vi "svfa_Check Data Valid [Nx1 Dual FFT].vi"(0 "stimulus signal X [EUx]":waveform(dbl), 1 "response signals Y [EUy]":waveform(dbl)[](array[waveform]), 2 "window":T3=1 items=["None"=0, "Hanning"=1, "Hamming"=2, "Blackman-Harris"=3, "Exact Blackman"=4, "Blackman"=5, "Flat Top"=6, "4 Term B-Harris "=7, "7 Term B-Harris"=8, "Low Sidelobe"=9, "Force - Exponential"=10, "Blackman Nuttall"=11, "Triangle"=30, "Bartlett-Hanning"=31, "Bohman"=32, "Parzen"=33, "Welch"=34, "Kaiser"=60, "Dolph-Chebyshev"=61, "Gaussian"=62], 3 "force/exp settings":T2={"force window [%]"=50.0, "exp window [%]"=10.0} {"exp window [%]" min=0.0 max=100.0 format="%.2f"; "force window [%]" min=0.0 max=100.0 format="%.2f"}, 4 "averaging parameters":T5={"averaging mode"=enum."No averaging", "weighting mode"=enum."Linear", "number of averages"=10, "linear mode"=enum."Auto restart"}, 5 "error in (no error)":errorcluster, 7 "processing control in":T4(ring), 8 "restart averaging (F)":bool, 9 "FRF mode":enum16{"H1", "H2", "H3"}(ring), 10 "measurement":T1(ring)=enum."Frequency response") -> (11 "dup FRF mode":enum16{"H1", "H2", "H3"}(ring), 13 "processing control out":T4(ring), 14 "dup stimulus signal X [EUx]":waveform(dbl), 15 "dup response signals Y [EUy]":waveform(dbl)[](array[waveform]), 16 "window":T3=1 items=["None"=0, "Hanning"=1, "Hamming"=2, "Blackman-Harris"=3, "Exact Blackman"=4, "Blackman"=5, "Flat Top"=6, "4 Term B-Harris "=7, "7 Term B-Harris"=8, "Low Sidelobe"=9, "Force - Exponential"=10, "Blackman Nuttall"=11, "Triangle"=30, "Bartlett-Hanning"=31, "Bohman"=32, "Parzen"=33, "Welch"=34, "Kaiser"=60, "Dolph-Chebyshev"=61, "Gaussian"=62], 17 "dup force/exp settings":T2={"force window [%]"=50.0, "exp window [%]"=10.0} {"exp window [%]" min=0.0 max=100.0 format="%.2f"; "force window [%]" min=0.0 max=100.0 format="%.2f"}, 18 "dup averaging parameters":T5={"averaging mode"=enum."No averaging", "weighting mode"=enum."Linear", "number of averages"=10, "linear mode"=enum."Auto restart"}, 19 "error out":errorcluster)   [LabVIEW 2017]
uses:
  <vilib>/addons/_NISVFA/_Shared subVIs/Controls/svc_Window [Dual FFT].ctl
  <vilib>/addons/_NISVFA/_Shared subVIs/Common/svc_Check for Waveform Parameter Continuity (N Ch).vi
  <vilib>/addons/_NISVFA/_Shared subVIs/Common/svc_Check for Waveform Parameter Continuity (1 Ch).vi
  <vilib>/addons/_NISVFA/_Shared subVIs/Common/svc_Check for Waveform Parameter Continuity (no state).vi
  <vilib>/addons/_NISVFA/_Shared subVIs/Common/svc_Get SV Channel Info.vi
  <vilib>/addons/_NISVFA/_Shared subVIs/Common/svc_Check dt for Equal Sample Rates.vi
  <vilib>/addons/_NISVFA/_Shared subVIs/Common/svc_Engineering Units to Unit Label.vi
  <vilib>/addons/_NISVFA/_Shared subVIs/Common/svc_Unit Label to Engineering Units.vi
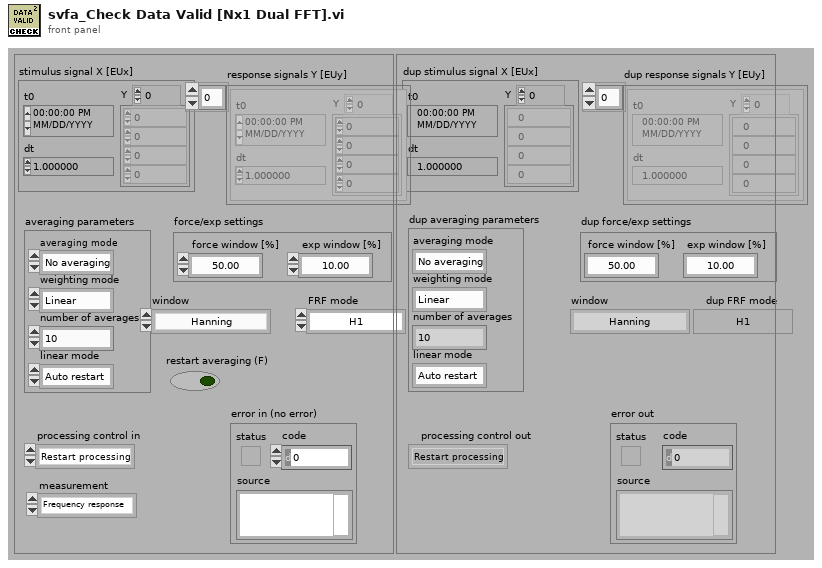
[diagram p1: front panel]
types:
  T1 = enum16{"Cross spectrum", "Frequency response", "Coherent output power"}
  T2 = cluster{"force window [%]":dbl, "exp window [%]":dbl}
  T3 = typedef "svc_Window [Dual FFT].ctl" = u32
  T4 = enum16{"Restart processing", "Continue processing", "Skip processing"}
  T5 = cluster{"averaging mode":enum16{"No averaging", "Vector averaging", "RMS averaging", "Peak hold"}, "weighting mode":enum16{"Linear", "Exponential"}, "number of averages":u32, "linear mode":enum16{"One shot", "Auto restart"}}
  T6 = cluster{"dt equal":bool, "array length equal":bool, "number channels change":bool}
  T7 = cluster{"dt":bool, "t0 continuity":bool, "array length":bool, "channel info":bool, "name":bool}
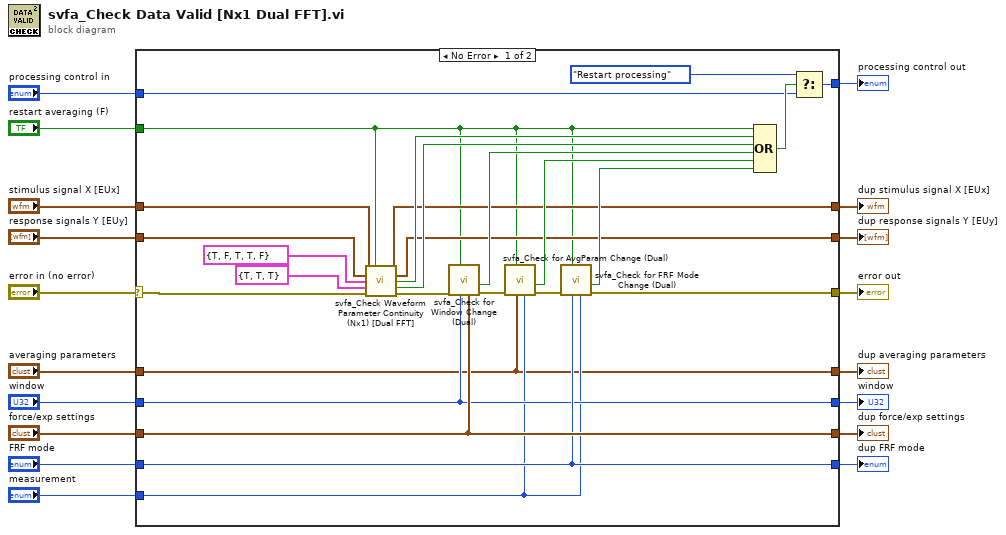
[diagram p0: block diagram]
diagram:
  n1 = case shown="No Error" "error in (no error)" {
    selector: "error in (no error)" -> [w23 w52]
    tunnel: [w21 w52] -> w18
    tunnel: "stimulus signal X [EUx]" -> [w25 w51]
    tunnel: [w24 w51] -> w16
    tunnel: "response signals Y [EUy]" -> [w27 w50]
    tunnel: [w26 w50] -> w14
    tunnel: "restart averaging (F)" -> [w22 _]
    tunnel: "processing control in" -> [w35 w47]
    tunnel: "FRF mode" -> [w42 w49]
    tunnel: "averaging parameters" -> [w32 w46]
    tunnel: "window" -> [w37 w45]
    tunnel: "force/exp settings" -> [w43 w48]
    tunnel: [w42 w49] -> w6
    tunnel: [w43 w48] -> w5
    tunnel: [w40 w47] -> w4
    tunnel: [w32 w46] -> w3
    tunnel: [w37 w45] -> w2
    tunnel: "measurement" -> [w33 _]
    frame No Error {
      n2 = call <vilib>:"svfa_Check Waveform Parameter Continuity (Nx1) [Dual FFT].vi"("stimulus signal X [EUx]"=w25, "restart averaging (F)"=w22, "response signals Y [EUy]"=w27, "checks for channel parameter change"=T7 {"dt"=TRUE, "t0 continuity"=FALSE, "array length"=TRUE, "channel info"=TRUE, "name"=FALSE}, "checks for multichannel parameters"=T6 {"dt equal"=TRUE, "array length equal"=TRUE, "number channels change"=TRUE}, "error in"=w23) -> ("dup stimulus signal X [EUx]"=w24:waveform(dbl), "dup response signals Y [EUy]"=w26:waveform(dbl)[], "waveform parameter changed"=w29:bool, "multichannel parameter changed"=w28:bool, "error out"=w30:errorcluster)  [unwired: 5 in]
      n3 = call <vilib>:"svfa_Check for Window Change (Dual).vi"("force/exp settings"=w43, "window"=w37, "restart averaging (F)"=w22, "error in (no error)"=w30) -> ("error out"=w36:errorcluster, "parameter has changed"=w39:bool)  [unwired: 6 in]
      n4 = call <vilib>:"svfa_Check for AvgParam Change (Dual).vi"("measurement"=w33, "averaging parameters"=w32, "restart averaging (F)"=w22, "error in (no error)"=w36) -> ("error out"=w34:errorcluster, "parameter has changed"=w31:bool)  [unwired: 6 in]
      n5 = call <vilib>:"svfa_Check for FRF Mode Change (Dual).vi"("measurement"=w33, "FRF mode"=w42, "restart"=w22, "error in (no error)"=w34) -> ("error out"=w21:errorcluster, "parameter has changed"=w38:bool)  [unwired: 6 in]
      n6 = Compound Arithmetic op=OR(w22, w29, w28, w39, w31, w38) -> (w41:bool)
      n7 = Select(t=T4."Restart processing", s=w41, f=w35) -> (s? t:f=w40:T4)
    }
    frame Error {
    }
  }
  "dup stimulus signal X [EUx]" <- w16
  "error out" <- w18
  "dup response signals Y [EUy]" <- w14
  "dup averaging parameters" <- w3
  "processing control out" <- w4
  "window" <- w2
  "dup force/exp settings" <- w5
  "dup FRF mode" <- w6
